vi "GET CONTROLLER VALUES.vi"(8 "error in (no error)":errorcluster, 10 "controller\nrefnum name":string) -> (0 "error out":errorcluster, 3 "controller out":T1)   [LabVIEW 2023]
uses:
  ctrl defs/ctrl controllers.ctl
  <vilib>/Rock Robotics/WPI/Utilities/WPI_GetSetVariantRefNum.vi
  <vilib>/Rock Robotics/Network Tables/NT Write Integer Array.vi
  <vilib>/Rock Robotics/Network Tables/NT Write Boolean Array.vi
  <vilib>/Rock Robotics/Network Tables/NT Write Numeric Array.vi
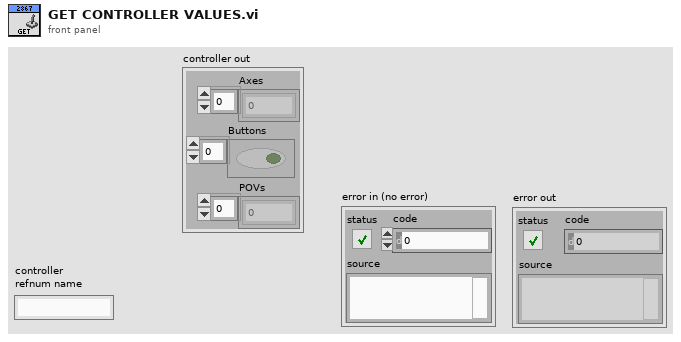
[diagram p1: front panel]
types:
  T1 = typedef "ctrl controllers.ctl" = cluster{"Axes":dbl[], "Buttons":bool[], "POVs":i16[]}
  T2 = typedef "WPI_JoystickDevRef.ctl" = cluster{"Device":T3}
  T3 = typedef "WPI_JoystickDeviceEnum.ctl" = enum16{"USB 0", "USB 1", "USB 2", "USB 3", "USB 4", "USB 5"}
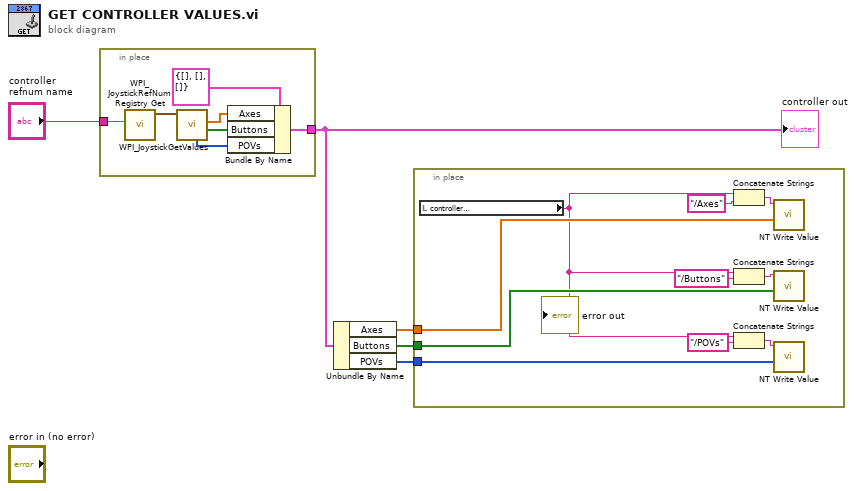
[diagram p0: block diagram]
diagram:
  n1 = in-place {
    in-place-border: "controller\nrefnum name" -> [w7]
    in-place-border: [w6] -> w4
    n2 = call <vilib>:"WPI_JoystickRefNum Registry Get.vi"("refnum name"=w7) -> ("JoystickDevRef"=w9:T2)  [unwired: 1 in, 9 out]
    n3 = call <vilib>:"WPI_JoystickGetValues.vi"("JoystickDevRef"=w9) -> ("Buttons"=w12:bool[], "Axes"=w11:dbl[], "POVs"=w8:i16[])  [unwired: 6 in, 2 out]
    n4 = Bundle By Name(cluster=T1 {"Axes"=[], "Buttons"=[], "POVs"=[]} ("controller in"), "Axes"=w11, "Buttons"=w12, "POVs"=w8) -> (w6:T1)
  }
  "controller out" <- w4
  n5 = Unbundle By Name(w4) -> ("Axes"=w3:dbl[], "Buttons"=w2:bool[], "POVs"=w1:i16[])
  n6 = in-place {
    in-place-border: w3 -> [w16]
    in-place-border: w2 -> [w15]
    in-place-border: w1 -> [w14]
    n7 = local read "controller\nrefnum name"() -> (w13:string)
    n8 = Concatenate Strings(w13, "/Axes" ("Name")) -> (w19:string)
    n9 = Concatenate Strings(w13, "/Buttons" ("Name")) -> (w20:string)
    n10 = Concatenate Strings(w13, "/POVs" ("Name")) -> (w17:string)
    n11 = call-poly <vilib>:"NT Write Value.vi"("value"=w16, "name"=w19) -> ()  [unwired: 9 in, 1 out]
    n12 = call-poly <vilib>:"NT Write Value.vi"("value"=w15, "name"=w20) -> ()  [unwired: 9 in, 1 out]
    n13 = call-poly <vilib>:"NT Write Value.vi"("value"=w14, "name"=w17) -> ()  [unwired: 9 in, 1 out]
  }
